vi "Read Websocket Message Broker Interface Ref.vi"(11 "Controller in":refnum<class "Controller.lvclass">) -> (2 "Stream Mediator.lvlib:Websocket Message Broker Interface Ref.lvclass":refnum<class "Websocket Message Broker Interface Ref.lvclass">, 3 "Controller out":refnum<class "Controller.lvclass">)   [LabVIEW 2016]
uses:
  <userlib>/Common Components/Controller/Controller.lvclass
  C:/Program Files (x86)/National Instruments/LabVIEW 2016/vi.lib/ActorFramework/Actor/Actor.lvclass
  <vilib>/Composed Systems/Stream/Mediator/Classes/Websocket Message Broker Interface Ref/Websocket Message Broker Interface Ref.lvclass
  C:/Program Files (x86)/National Instruments/LabVIEW 2016/vi.lib/Composed Systems/Stream/Mediator/Classes/Message Broker Interface Ref/Message Broker Interface Ref.lvclass
  C:/Program Files (x86)/National Instruments/LabVIEW 2016/vi.lib/Composed Systems/Stream/Mediator/Classes/Message Broker Interface/Message Broker Interface.lvclass
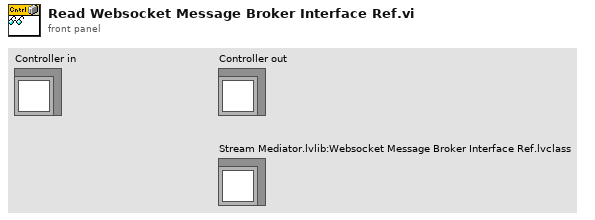
[diagram p1: front panel]
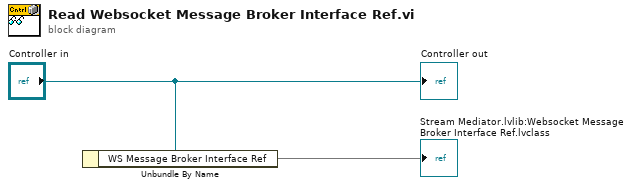
[diagram p0: block diagram]
diagram:
  n1 = Unbundle By Name("Controller in") -> ("WS Message Broker Interface Ref"=→"Stream Mediator.lvlib:Websocket Message Broker Interface Ref.lvclass")
  "Controller out" <- "Controller in"
